vi "CalculateTotalNumberFreezedDroplets.vi"() -> ()   [LabVIEW 2013]
panel:
  out "FreezeBoolArray":dbl[](array[numeric])
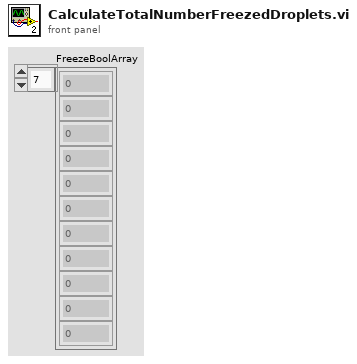
[diagram p1: front panel]
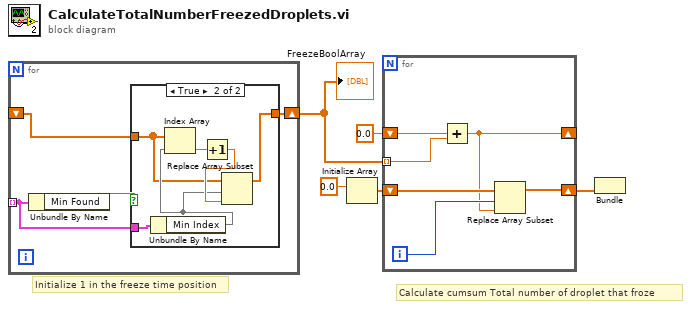
[diagram p0: block diagram]
diagram:
  # "Calculate cumsum Total number of droplet that froze"
  # "Initialize 1 in the freeze time position"
  n1 = for {
    tunnel: _ -> [w10] mode=indexing
    shift-right: [w8] -> w2
    shift-left: _ -> [w9]
    n2 = Unbundle By Name(w10) -> ("Min Found"=w11)
    n3 = case shown="True" w11 {
      tunnel: w10 -> [_ w18]
      tunnel: w9 -> [w12 w14]
      tunnel: [w12 w13] -> w8
      frame False {
      }
      frame True {
        n4 = Unbundle By Name(w18) -> ("Min Index"=w15)
        n5 = Index Array(array=w14, index=w15) -> (element=w17:dbl)
        n6 = Increment(x=w17) -> (x+1=w16:dbl)
        n7 = Replace Array Subset(array=w14, new element=w16, index=w15) -> (w13:dbl[])
      }
    }
  }
  "FreezeBoolArray" <- w2
  n8 = Initialize Array(0.0 ("element")) -> (w5:dbl[], w4:i32)
  n9 = for {
    tunnel: w2 -> [w23] mode=indexing
    shift-right: [w19] -> w7
    shift-left: w5 -> [w22]
    shift-right: [w20] -> _
    shift-left: 0.0 -> [w24]
    i -> [w21]
    n10 = Add(x=w24, y=w23) -> (x+y=w20:dbl)
    n11 = Replace Array Subset(array=w22, new element=w20, index=w21) -> (w19:dbl[])
  }
  n12 = Bundle(w7) -> (w1)  [unwired: 1 in, 1 out]
